vi "Compatibility Trigger Each Line From Encoder.vi"() -> ()   [LabVIEW 2023]
doc: "The Compatibility Trigger Each Line From Encoder example uses the Phase A & B pins from an encoder to trigger the acquisition of each image line. Because the encoder frequency is generally higher than the desired line rate, use the <B>Divide Factor</B> to adjust the <B>Scaled Encoder</B> signal frequency to match that of the desired line rate. The encoder hardware on IMAQ devices is designed to accomodate backlash, so the <B>Scaled Encoder</B> signal will only pulse for cumulative forward movement of the encoder itself.\n\nThis example requires a linescan camera with an IMAQ device that supports encoder hardware. \n\nThis example uses the IMAQdx driver to interface with a Camera Link frame grabber. It uses the NI-IMAQdx Compatibility for NI-IMAQ API to facilitate migration between the two drivers. The NI-IMAQdx VIs are drop-in replacements to existing NI-IMAQ VIs."
uses:
  <vilib>/vision/driver/NI_Vision_Acquisition_Software.lvlib
  <resource>/objmgr/imaqdx.rc
panel:
  in  "Camera Name":refnum<k21> caption="IMAQdx Session"
  in  "Encoder Parameters":T1={"Divide Factor"=10, "Phase A Polarity"=0, "Phase B Polarity"=0, "Phase A & B Filter"=FALSE} {"Phase B Polarity" items=["Active High", "Active Low"]; "Phase A Polarity" items=["Active High", "Active Low"]}
  in  "Stop":bool
  out "Image":T2(plugin-control)
  out "Last Valid Buffer":u32
  # "Overview: Demonstrates how to trigger the acquisition of each image line from an encoder. \nRequirements: Vision Acquisition Software, PCIe-1427, PCIe-1433, PXIe-1435, or PCIe-1437 frame grabber, Linescan camera.\nInstructions: \n1. Select the Camera Name.\n2. Run the VI.\n3. Send encoder signals to the frame grabber to trigger each line of the linescan camera to be acquired."
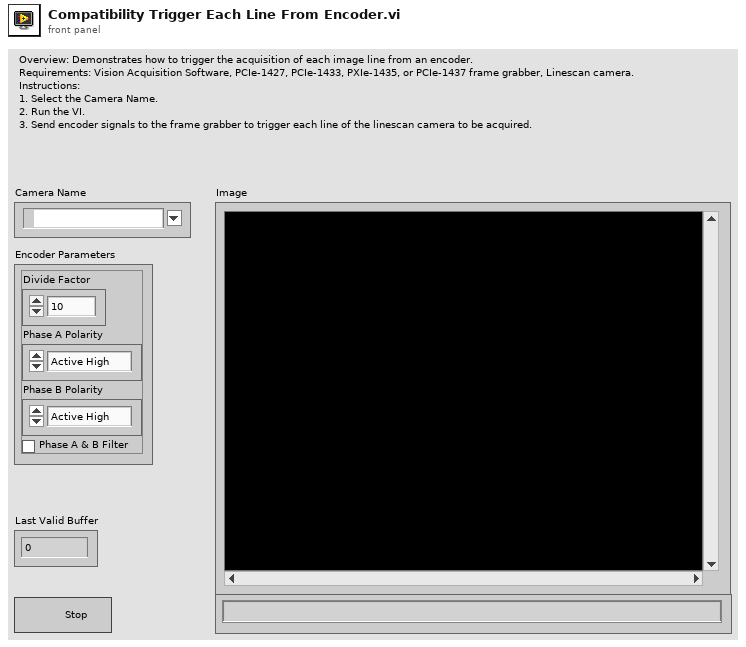
[diagram p1: front panel]
types:
  T1 = cluster{"Divide Factor":u32, "Phase A Polarity":u32, "Phase B Polarity":u32, "Phase A & B Filter":bool}
  T2 = typedef "IMAQ Image.ctl" = refnum<image>
  T3 = typedef "IMAQdx.ctl" = refnum<k21>
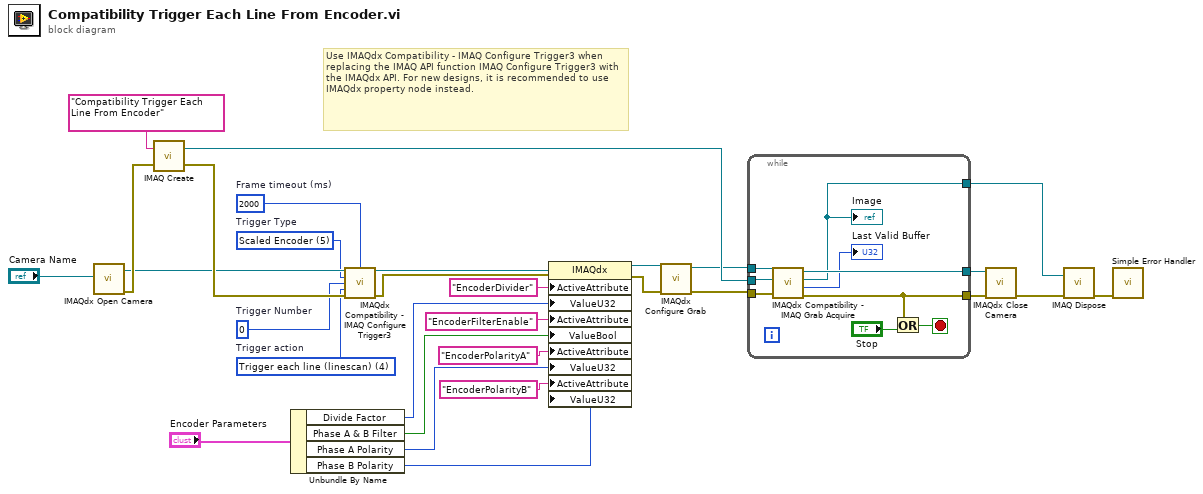
[diagram p0: block diagram]
diagram:
  w1 = u32 0  # Trigger Number
  w20 = u32 5 items=["External"=0, "RTSI"=1, "ISO In"=2, "Scaled Encoder"=5]  # Trigger Type
  w21 = u32 4 items=["Disabled", "Trigger start of acquisition", "Trigger start of each buffer list", "Trigger each buffer", "Trigger each line (linescan)"]  # Trigger action
  w22 = u32 2000  # Frame timeout (ms)
  # "Use IMAQdx Compatibility - IMAQ Configure Trigger3 when replacing the IMAQ API function IMAQ Configure Trigger3 with the IMAQdx API. For new designs, it is recommended to use IMAQdx property node instead."
  n1 = call <vilib>:"IMAQdx Open Camera.vi"("Session In"="Camera Name") -> ("error out"=w25:errorcluster, "Session Out"=w23:T3)  [unwired: 9 in]
  n2 = call "IMAQ Create"("Image Name"="Compatibility Trigger Each Line From Encoder" ("format string"), "error in (no error)"=w25) -> ("New Image"=w27:T2, "error out"=w24:errorcluster)  [unwired: 2 in, 1 out]
  n3 = Unbundle By Name("Encoder Parameters") -> ("Divide Factor"=w18:u32, "Phase A & B Filter"=w17:bool, "Phase A Polarity"=w16:u32, "Phase B Polarity"=w15:u32)
  n4 = call <vilib>:"IMAQdx Compatibility - IMAQ Configure Trigger3.vi"("Session In"=w23, "Frame timeout (ms)"=w22, "Type"=w20, "Line Number"=w1, "Action"=w21, "error in (no error)"=w24) -> ("Session Out"=w19:T3, "error out"=w7:errorcluster)  [unwired: 8 in]
  n5 = property class="IMAQdx"(reference=w19, error in=w7, "ActiveAttribute"="EncoderDivider", "ValueU32"=w18, "ActiveAttribute"="EncoderFilterEnable", "ValueBool"=w17, "ActiveAttribute"="EncoderPolarityA", "ValueU32"=w16, "ActiveAttribute"="EncoderPolarityB", "ValueU32"=w15) -> (reference out=w14:T3, error out=w13:errorcluster)
  n6 = call <vilib>:"IMAQdx Configure Grab.vi"("error in"=w13, "Session In"=w14) -> ("error out"=w11:errorcluster, "Session Out"=w12:T3)  [unwired: 8 in]
  n7 = while {
    tunnel: [w34] -> w10
    tunnel: [w31] -> w9
    tunnel: w27 -> [w37]
    tunnel: [w33] -> w26
    tunnel: w12 -> [w36]
    tunnel: w11 -> [w35]
    stop <- w39 stop-if-true
    n8 = call <vilib>:"IMAQdx Compatibility - IMAQ Grab Acquire.vi"("error in (no error)"=w35, "Image In"=w37, "Session In"=w36) -> ("error out"=w31:errorcluster, "Acquired Buffer Number"=→"Last Valid Buffer":u32, "Image Out"=w33:T2, "Session Out"=w34:T3)  [unwired: 5 in]
    "Image" <- w33
    n9 = Or(x=w31, y="Stop") -> (x .or. y?=w39:bool)
  }
  n10 = call <vilib>:"IMAQdx Close Camera.vi"("error in"=w9, "Session In"=w10) -> ("error out"=w8:errorcluster)  [unwired: 9 in]
  n11 = call "IMAQ Dispose"("Image"=w26, "error in (no error)"=w8) -> ("error out"=w30:errorcluster)  [unwired: 1 in, 3 out]
  n12 = call <vilib>:"Simple Error Handler.vi"("error in (no error)"=w30) -> ()  [unwired: 1 in, 8 out]
